vi "Ctrls_ReinitializeToDefault.vi"(7 "TAG":string, 8 "error in (no error)":errorcluster, 10 "DB Ref":T1, 11 "String":string) -> (0 "error out":errorcluster)   [LabVIEW 2017, in "tagdb-UIStateExpr Operations.lvlib"]
uses:
  tagdb-UIStateExpr Operations.lvlib
  <userlib>/_NEVSTOP/TagDB/Typedef/TagDB.ctl
  36e5cb1f-7625-4e24-8fa4-500bcd356289.vi
  36e5cb1f-7625-4e24-8fa4-500bcd356289.vi/1b47866c-8e2d-43a7-815f-8cf18635e5a1.vi
  <userlib>/_NEVSTOP/TagDB/_Support/Change Detector/TagDB dbChanged.vi
  <userlib>/_NEVSTOP/TagDB/_Support/Error/_Clear Errors.vi
  36e5cb1f-7625-4e24-8fa4-500bcd356289.vi/1b47866c-8e2d-43a7-815f-8cf18635e5a1.vi/29b2ea6d-6d7f-4e4a-ad31-a5cb760462c7.vi
  <userlib>/_NEVSTOP/TagDB/API/TagDB-Status.vi
  <userlib>/_NEVSTOP/TagDB/_Support/Change Detector/TagDB ChangeFlag.vi
  <userlib>/_NEVSTOP/TagDB/_Support/DataAccess/_NameCacher.vi
  <userlib>/_NEVSTOP/TagDB/_Support/Error/_[error50002]Invalid DataType.vi
  <userlib>/_NEVSTOP/TagDB/_Support/Error/_[error50000]Invalid DB REF.vi
  <userlib>/_NEVSTOP/TagDB/_Support/DataAccess/TagDB Ref to DVR.vi
  <userlib>/_NEVSTOP/TagDB/_Support/URL/TRIM-BOTH-SPACE.vi
  <userlib>/_NEVSTOP/TagDB/_Support/Error/_Build Error Cluster.vi
  <userlib>/_NEVSTOP/TagDB/TagDB.lvlib
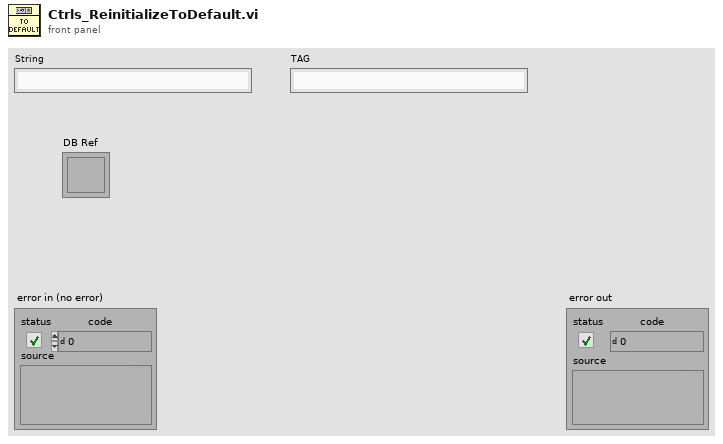
[diagram p1: front panel]
types:
  T1 = typedef "TagDB.lvlib/TagDB.ctl" = refnum<k1>
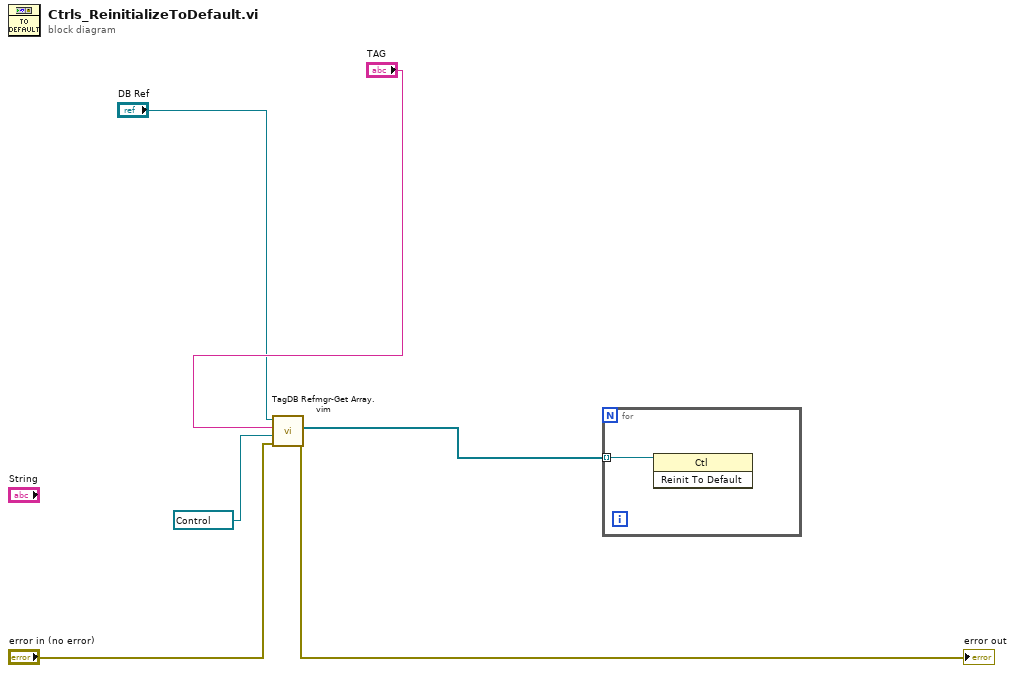
[diagram p0: block diagram]
diagram:
  n1 = call "TagDB Refmgr-Get Array.vim"("error in (no error)"="error in (no error)", "Type"=refnum<vi> refnum, "RegExp"="TAG", "DB Ref"="DB Ref") -> ("error out"=→"error out":errorcluster, "References"=w4:refnum<vi>[])  [unwired: 4 in, 2 out]
  n2 = for {
    tunnel: w4 -> [w7] mode=indexing
    n3 = invoke class="Ctl" method="Reinit To Default"(reference=w7) -> ()  [unwired: 2 in, 3 out]
  }
